vi "QMH Destroy Queue.vi"(8 "error in (no error)":errorcluster, 11 "queue in":refnum<queue>) -> (0 "error out":errorcluster, 2 "Remaining Events":string[](array[string]), 3 "queue name":string)   [LabVIEW 2011]
doc: "Release the reference to the event queue and return any remaing events."
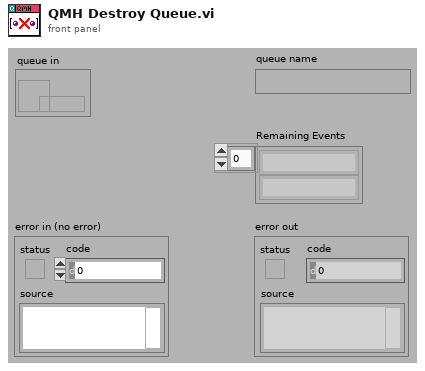
[diagram p1: front panel]
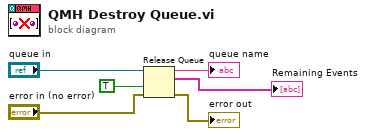
[diagram p0: block diagram]
diagram:
  n1 = Release Queue(queue="queue in", force destroy? (F)=TRUE, error in (no error)="error in (no error)") -> (queue name=→"queue name":string, remaining elements=→"Remaining Events":string[], error out=→"error out":errorcluster)
